vi "Prompt for App Instance.vi"(8 "error in (no error)":errorcluster, 10 "Calling VI in":refnum<vi>, 11 "App Instances":T1[](array[typedef])) -> (0 "error out":errorcluster, 2 "OK?":bool, 3 "App Ref":refnum<vi>)   [LabVIEW 2020, in "MacroAssert.lvlib"]
doc: "Displays a window to select the application instance to connect to."
uses:
  MacroAssert.lvlib
  FaKI State Machine/FaKI State Machine.lvlib
  CTLs/FGV Actions.ctl
  Custom Errors/Custom Errors.lvlib
  <vilib>/Utility/miscctls.llb/LVComboBoxStrsAndValuesArrayTypeDef.ctl
  CTLs/App Instance.ctl
  <userlib>/_MGI/Application Control/MGI Gray if/MGI Gray if False.vi
panel:
  in  "Project":string(combo)
  in  "App Instance":string(combo)
  in  "OK":bool
  in  "Exit":bool
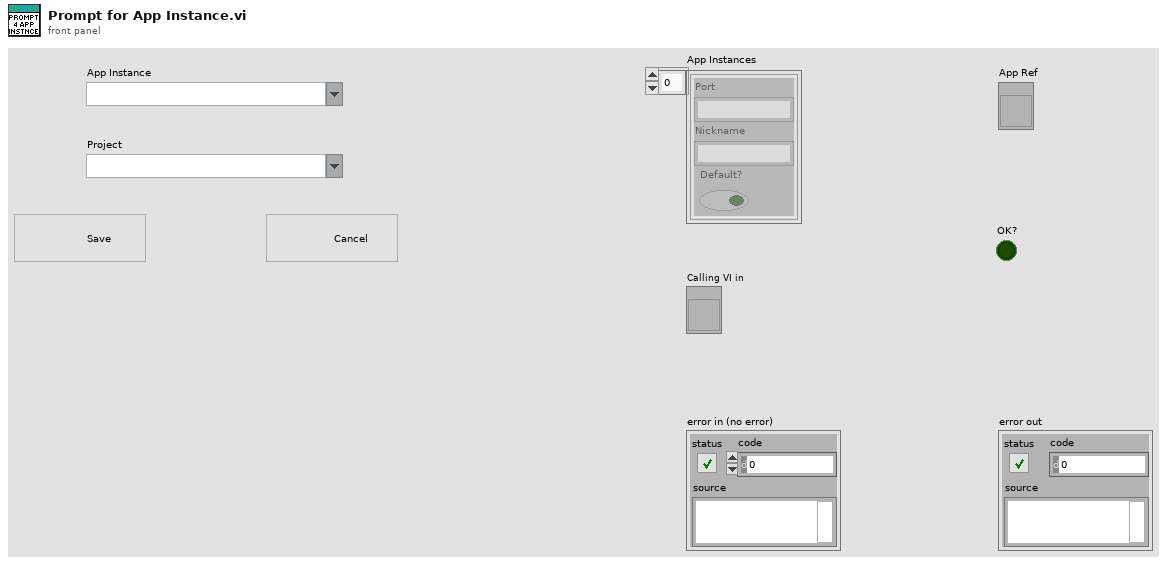
[diagram p1: front panel]
types:
  T1 = typedef "MacroAssert.lvlib/App Instance.ctl" = cluster{"Port":string, "Nickname":string, "Default?":bool}
  T2 = enum32{"Invalid", "Standard", "Closed", "Hidden", "Minimized", "Maximized"}
  T3 = enum32{"invalid app kind", "Development System", "Run Time System", "Student Edition", "Embedded LabVIEW", "Evaluation", "Custom"}
  T4 = typedef "LVComboBoxStrsAndValuesArrayTypeDef.ctl" = cluster{"String":string, "Value":string}[]
  T5 = typedef "MacroAssert.lvlib/FGV Actions.ctl" = enum16{"Read", "Write"}
  T6 = cluster{"Core":cluster{"Current VI Reference":refnum<vi>, "Close Panel on Exit?":bool}, "App Instances":T1[], "Current App":T1, "Current Proj":path, "App Ref":refnum<vi>, "Projects":cluster{"Name":string, "Path":path}[], "OK?":bool}
  T7 = cluster{"Current VI Reference":refnum<vi>, "Close Panel on Exit?":bool}
  T8 = enum8{"Enabled", "Disabled", "Disabled and Grayed Out"}
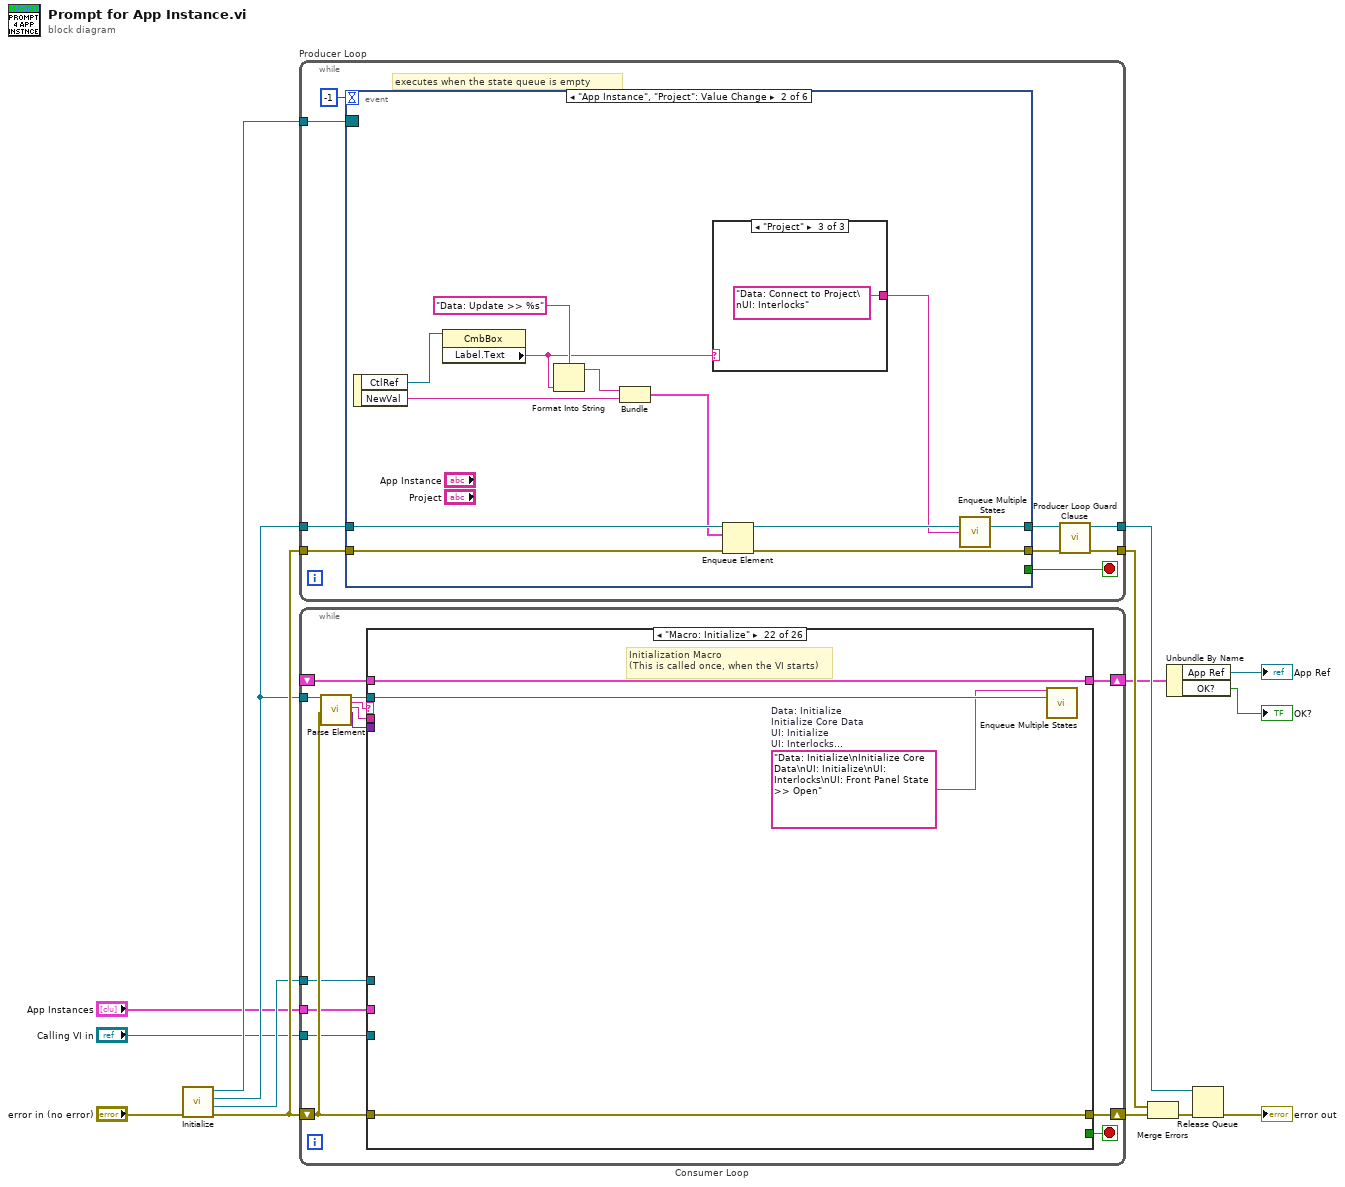
[diagram p0: block diagram]
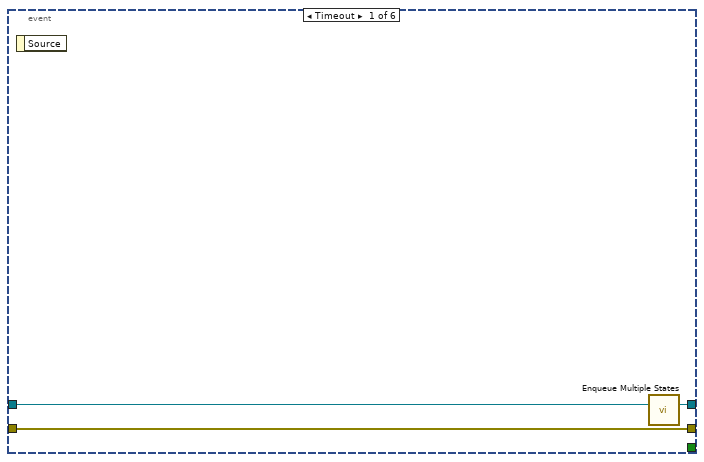
[diagram p2: hidden frame]
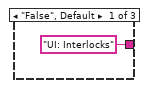
[diagram p3: hidden frame]
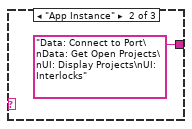
[diagram p4: hidden frame]
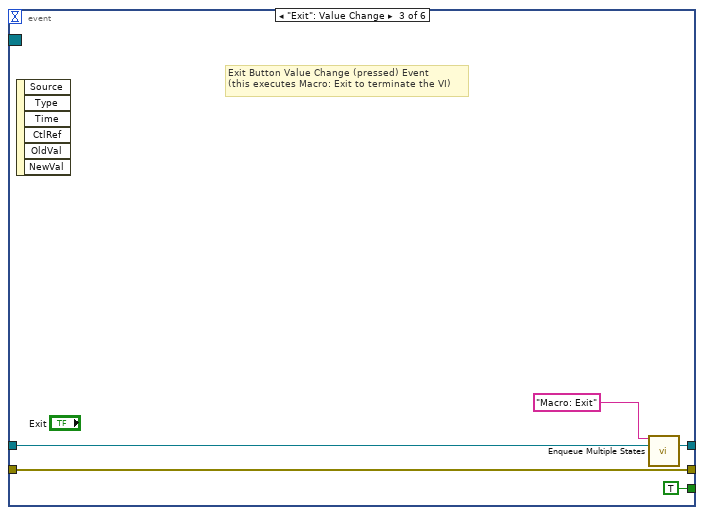
[diagram p5: hidden frame]
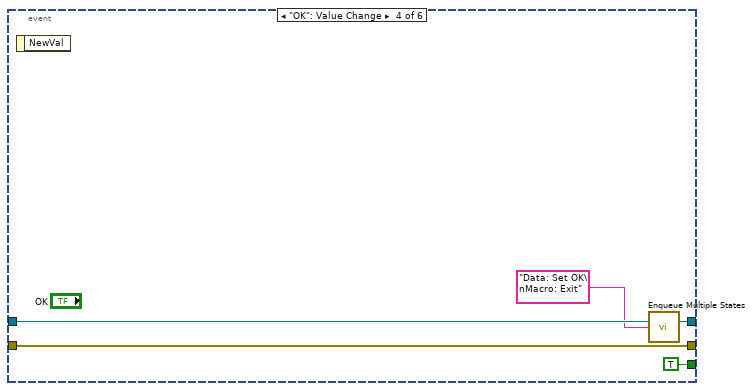
[diagram p6: hidden frame]
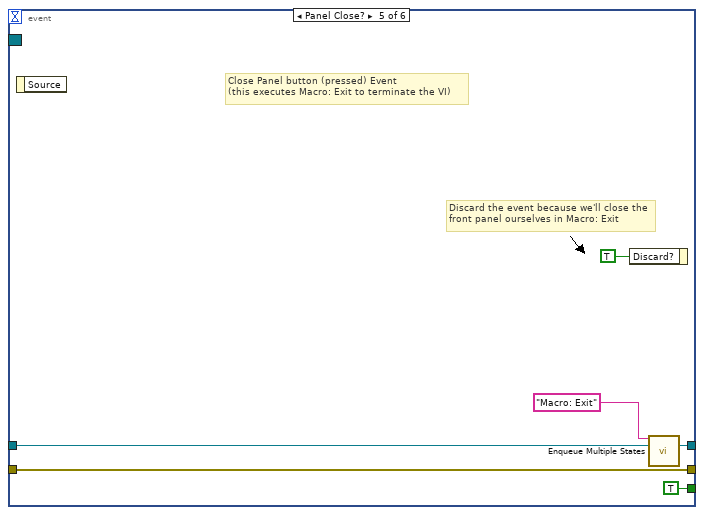
[diagram p7: hidden frame]
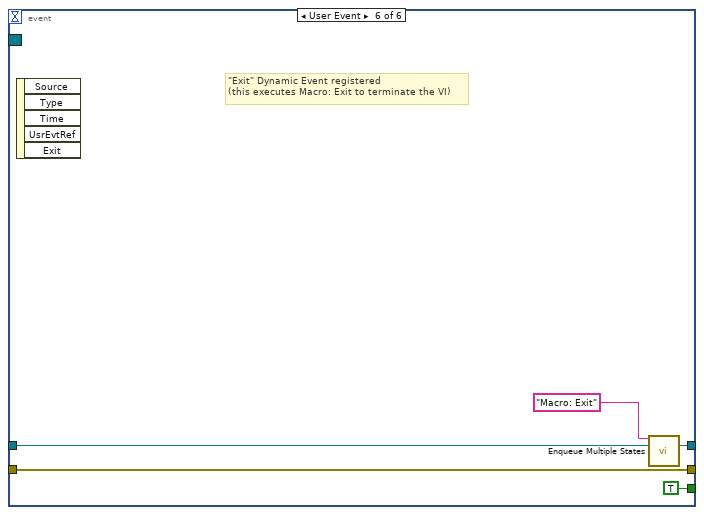
[diagram p8: hidden frame]
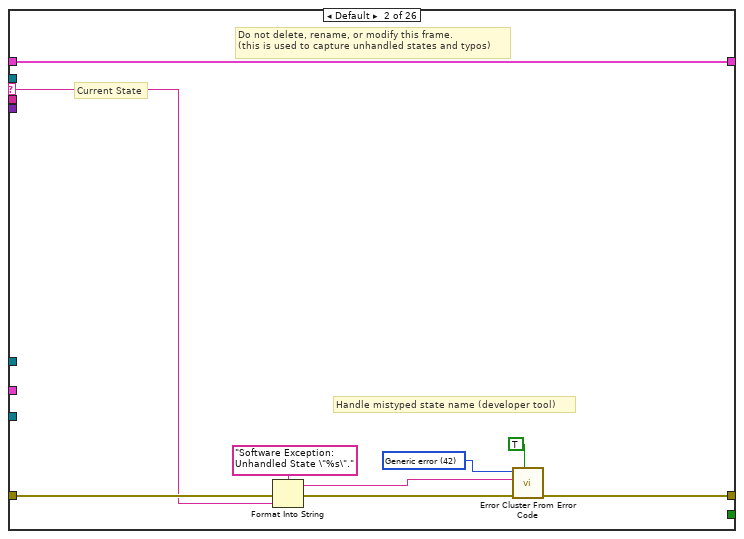
[diagram p10: hidden frame]
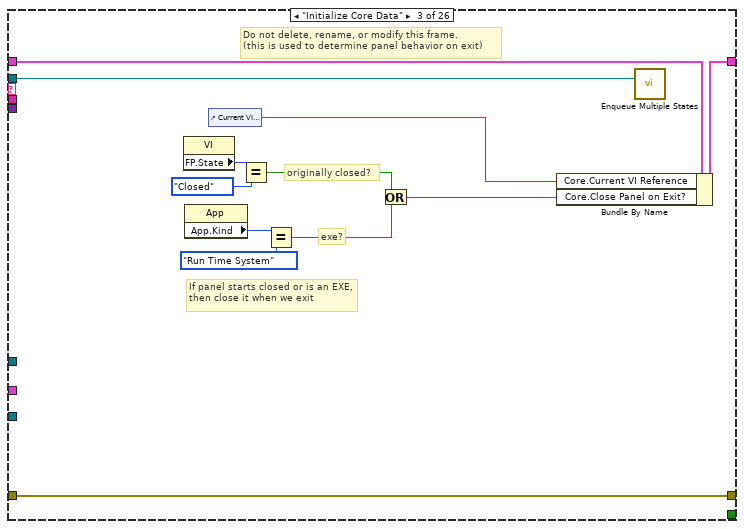
[diagram p11: hidden frame]
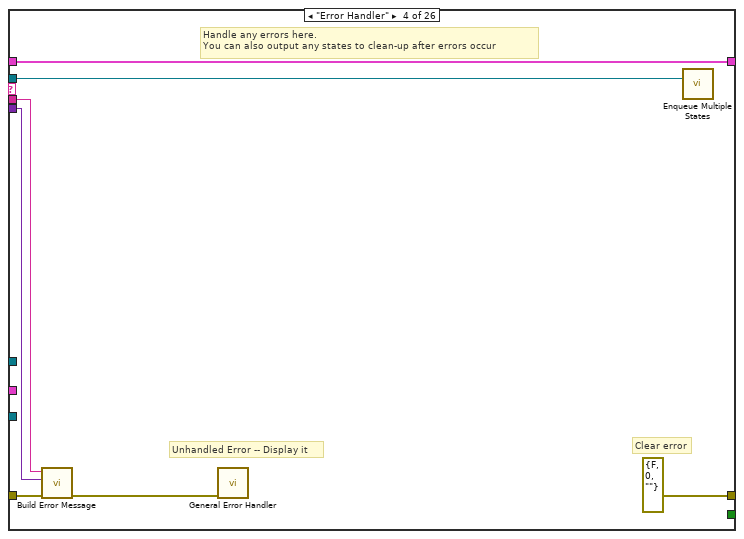
[diagram p12: hidden frame]
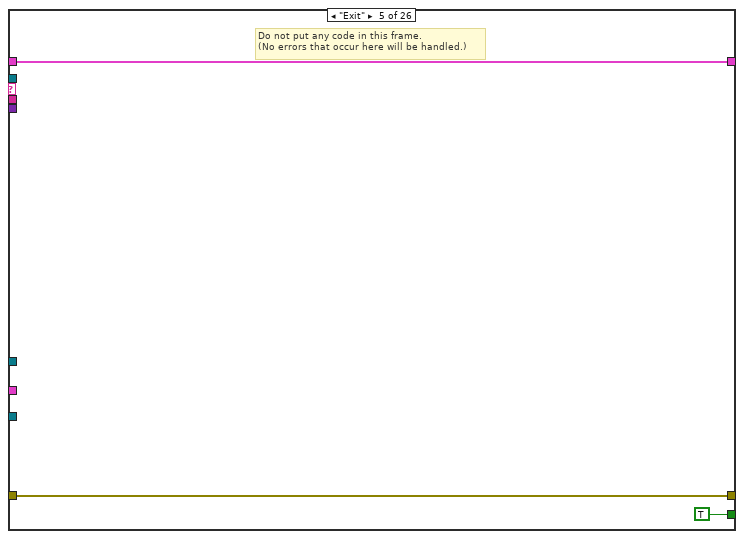
[diagram p13: hidden frame]
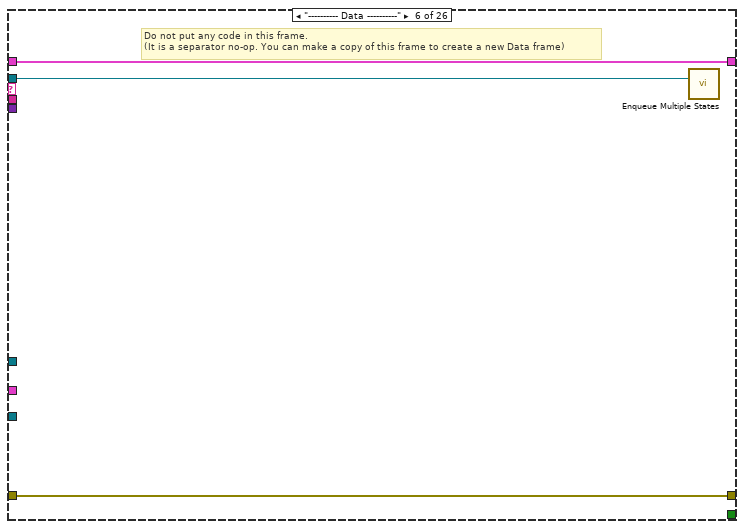
[diagram p14: hidden frame]
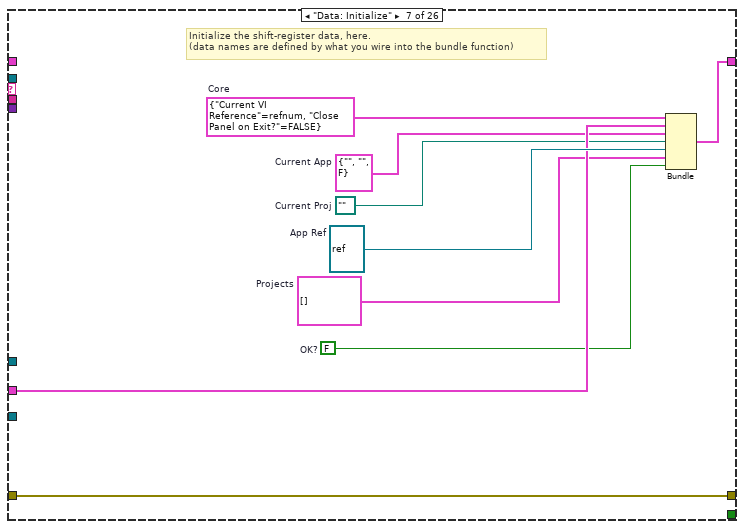
[diagram p15: hidden frame]
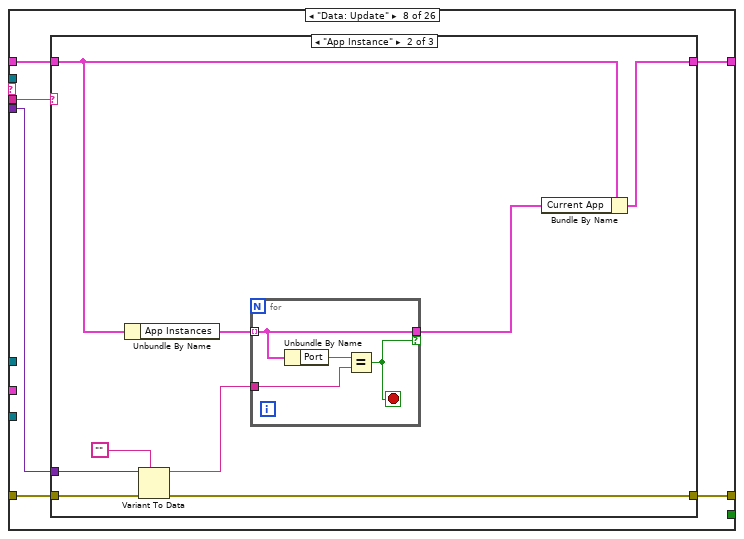
[diagram p16: hidden frame]
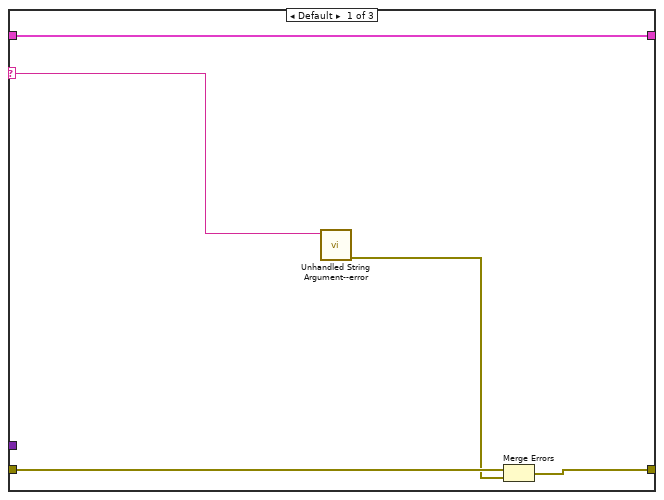
[diagram p17: hidden frame]
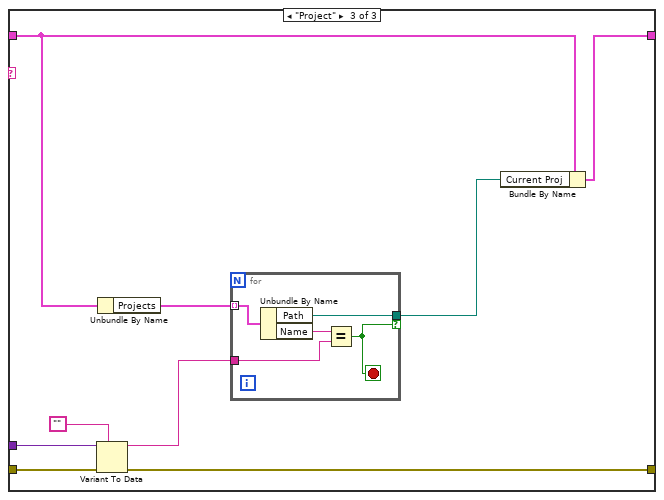
[diagram p18: hidden frame]
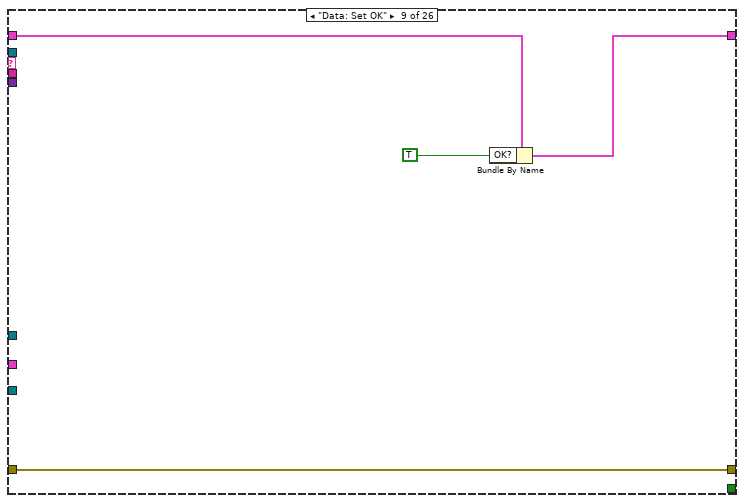
[diagram p19: hidden frame]
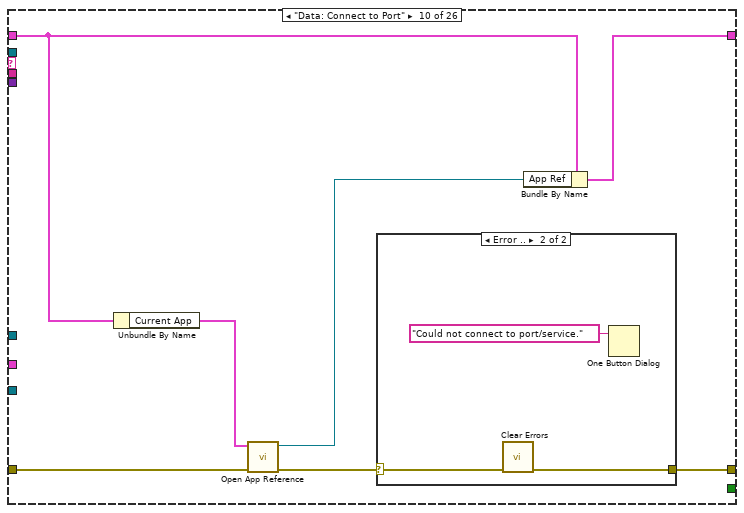
[diagram p20: hidden frame]
diagram:
  n1 = call "Initialize.vi"("error in (no error)"="error in (no error)") -> ("error out"=w11:errorcluster, "Exit Event"=w8:refnum<user-event>, "Queue"=w7:refnum<queue>, "Event Registration Refnum"=w6:refnum<event-registration>)  [unwired: 7 in]
  n2 = while "Producer Loop" {
    tunnel: w6 -> [w18]
    tunnel: w7 -> [w21]
    tunnel: [w19] -> w9
    tunnel: w11 -> [w24]
    tunnel: [w22] -> w14
    stop <- w16 stop-if-true
    # "executes when the state queue is empty"
    n3 = event shown="[1] \"App Instance\", \"Project\": Value Change" {
      selector: w18 -> [_ _ _ _ _ _]
      dyn-events: _ -> [_ _ _ _ _ _]
      timeout: -1 ("Timeout") -> [_ _ _ _ _ _]
      tunnel: [w27 w38 w47 w52 w58 w63] -> w23
      tunnel: w24 -> [w27 w39 w47 w52 w58 w63]
      tunnel: w21 -> [w25 w37 w46 w51 w57 w62]
      tunnel: [w26 w34 w45 w50 w56 w61] -> w20
      tunnel: [_ _ TRUE TRUE TRUE TRUE] -> w16
      event Timeout {
        n4 = event-data() -> ()  [unwired: 1 in, 1 out]
        n5 = call "Enqueue Multiple States.vi"("queue in"=w25) -> ("queue out"=w26:refnum<queue>)  [unwired: 14 in]
      }
      event "App Instance", "Project": Value Change {
        n6 = event-data() -> ("CtlRef"=w35:refnum<vi>, "NewVal"=w28:string)  [unwired: 1 in]
        n7 = property class="CmbBox"(reference=w35) -> ("Label.Text"=w30:string)  [unwired: 1 in, 2 out]
        n8 = Format Into String(format string="Data: Update >> %s", w30) -> (resulting string=w31:string)  [unwired: 2 in, 1 out]
        n9 = Bundle(w31, "NewVal"=w28) -> (w29:cluster{string, "NewVal":string})  [unwired: 1 in]
        n10 = case shown="\"Project\"" w30 {
          tunnel: ["UI: Interlocks" ("string") "Data: Connect to Port\nData: Get Open Projects\nUI: Display Projects\nUI: Interlocks" ("string") "Data: Connect to Project\nUI: Interlocks" ("string")] -> w33
          frame "False", Default {
          }
          frame "App Instance" {
          }
          frame "Project" {
          }
        }
        n11 = Enqueue Element(queue=w37, element=w29, error in (no error)=w39) -> (queue out=w36:refnum<queue>, error out=w38:errorcluster)  [unwired: 1 in, 1 out]
        n12 = call "Enqueue Multiple States.vi"("queue in"=w36, "State(s) at Back"=w33) -> ("queue out"=w34:refnum<queue>)  [unwired: 13 in]
      }
      event "Exit": Value Change {
        # "Exit Button Value Change (pressed) Event\n(this executes Macro: Exit to terminate the VI)"
        n13 = event-data() -> ()  [unwired: 1 in, 6 out]
        n14 = call "Enqueue Multiple States.vi"("State(s) at Front"="Macro: Exit", "queue in"=w46) -> ("queue out"=w45:refnum<queue>)  [unwired: 13 in]
      }
      event "OK": Value Change {
        n15 = event-data() -> ()  [unwired: 1 in, 1 out]
        n16 = call "Enqueue Multiple States.vi"("queue in"=w51, "State(s) at Back"="Data: Set OK\nMacro: Exit") -> ("queue out"=w50:refnum<queue>)  [unwired: 13 in]
      }
      event Panel Close? {
        # "Discard the event because we'll close the front panel ourselves in Macro: Exit"
        # "Close Panel button (pressed) Event\n(this executes Macro: Exit to terminate the VI)"
        n17 = event-data() -> ()  [unwired: 1 in, 1 out]
        n18 = event-data("Discard?"=TRUE) -> ()  [unwired: 1 in, 1 out]
        n19 = call "Enqueue Multiple States.vi"("State(s) at Front"="Macro: Exit", "queue in"=w57) -> ("queue out"=w56:refnum<queue>)  [unwired: 13 in]
      }
      event User Event {
        # "\"Exit\" Dynamic Event registered\n(this executes Macro: Exit to terminate the VI)"
        n20 = event-data() -> ()  [unwired: 1 in, 5 out]
        n21 = call "Enqueue Multiple States.vi"("State(s) at Front"="Macro: Exit", "queue in"=w62) -> ("queue out"=w61:refnum<queue>)  [unwired: 13 in]
      }
    }
    n22 = call "Producer Loop Guard Clause.vi"("error in (no error)"=w23, "queue in"=w20) -> ("error out"=w22:errorcluster, "queue out"=w19:refnum<queue>)  [unwired: 8 in]
  }
  n23 = while "Consumer Loop" {
    shift-right: [w69] -> w3
    shift-left: _ -> [w68]
    shift-right: [w76] -> w13
    shift-left: w11 -> [w75]
    tunnel: w7 -> [w74]
    tunnel: w8 -> [w72]
    tunnel: "App Instances" -> [w64]
    tunnel: "Calling VI in" -> [w71]
    stop <- w70 stop-if-true
    n24 = call "Parse Element.vi"("queue in"=w74, "error in (no error)"=w75) -> ("queue out"=w73:refnum<queue>, "State"=w67:string, "Arg"=w66:string, "Data"=w65:variant)  [unwired: 14 in]
    n25 = case shown="\"Macro: Initialize\"" w67 {
      selector: w67 -> [_ w79 _ _ _ _ _ _ _ _ _ _ _ _ _ _ _ _ _ _ _ _ _ _ _ _]
      tunnel: w73 -> [_ _ w97 w103 _ w111 _ _ _ _ _ _ _ _ _ _ _ _ _ _ _ w348 w358 _ _ w373]
      tunnel: w66 -> [_ _ _ w100 _ _ _ w125 _ _ _ _ _ _ _ _ w227 w235 _ _ _ _ _ _ _ _]
      tunnel: w68 -> [w77 w81 w92 w102 w108 w110 _ w124 w162 w165 w176 w188 w208 w212 w216 w225 w228 w236 w314 w340 w344 w347 w357 w360 w364 w372]
      tunnel: [w78 w86 w99 errorcluster {"status"=FALSE, "code"=0, "source"=""} ("error out") w109 w112 w121 w126 w163 w168 w180 w189 w210 w213 w217 w226 w229 w239 w318 w341 w345 w349 w359 w361 w365 w374] -> w76
      tunnel: w75 -> [w78 w85 w99 w105 w109 w112 w121 w127 w163 w170 w182 w190 w211 w213 w217 w226 w230 w240 w317 w341 w345 w349 w359 w361 w366 w375]
      tunnel: [_ _ _ _ TRUE _ _ _ _ _ _ _ _ _ _ _ _ _ _ _ _ _ _ _ _ _] -> w70
      tunnel: [w77 w81 w96 w102 w108 w110 w119 w122 w161 w166 w177 w187 w208 w212 w216 w225 w228 w236 w314 w340 w344 w347 w357 w360 w364 w372] -> w69
      tunnel: w65 -> [_ _ _ w101 _ _ _ w123 _ _ _ _ _ _ _ _ _ _ _ _ _ _ _ _ _ _]
      tunnel: w72 -> [_ _ _ _ _ _ _ _ _ _ _ _ _ _ _ _ _ _ _ _ _ _ _ _ _ _]
      tunnel: w64 -> [_ _ _ _ _ _ w117 _ _ _ _ _ _ _ _ _ _ _ _ _ _ _ _ _ _ _]
      tunnel: w71 -> [_ _ _ _ _ _ _ _ _ _ _ _ _ _ _ _ _ w237 _ _ _ _ _ _ _ _]
      frame "---------- Core ----------" {
        # "Do not put any code in this frame.\n(it is a separator no-op)"
      }
      frame Default {
        w83 = 42 items=["No error", "Argument error", "Memory is full", "Out of zone", "End of file", "File already open", "Generic file I/O error", "File not found", "File permission error", "Disk is full", "Duplicate path", "Too many files open", "System feature not enabled", "Resource file not found", "Cannot add resource", "Resource not found", "Image not found", "Image memory error", "Pen does not exist", "Config type invalid", "Config token not found", "Config parse error", "Config memory error", "Bad external code format", "Bad external code offset", "External code not present", "Null window", "Destroy window error", "Null menu", "Print aborted", "Bad print record", "Print driver error", "Windows error during printing", "Memory error during printing", "Print dialog error", "Generic print error", "Invalid device refnum", "Device not found", "Device parameter error", "Device unit error", "Cannot open device", "Device call aborted", "Generic error", "Cancelled by user", "Object ID too low", "Object ID too high", "Object not in heap", "Unknown heap", "Unknown object (invalid DefProc)", "Unknown object (DefProc not in table)", "Message out of range", "Invalid (null) method", "Unknown message", "Manager call not supported", "Bad address", "Network operation in progress", "Network operation timed out", "Connection is busy", "Network attribute not supported", "Network error", "Address in use", "System out of memory", "Connection aborted", "Connection refused", "Not connected", "Already connected", "Connection closed", "Initialization error (interapplication manager)", "Bad occurrence", "Wait on unbound occurrence handler", "Occurrence queue overflow", "Datalog type conflict", "Unused", "Unrecognized type (interapplication manager)", "Memory corrupt", "Failed to make temporary DLL", "Old CIN version", "Drag socket not found", "Failed to load drop-object", "Failed to register OLE object", "Failed to release OLE object", "Format specifier type mismatch", "Unknown format specifier", "Too few format specifiers", "Too many format specifiers", "Scan failed", "Newer CIN version", "Error converting to variant", "Runtime menu error", "Password tampered", "Variant attribute not found", "Incompatible variant data type", "Event data is not available", "Event Store is not present", "Occurrence is not found", "Event Queue is not created", "Event info is not available", "Refnum passed is NULL", "Error retrieving Class GUID", "Error retrieving CoClass GUID", "Error retrieving TypeLib GUID.", "Bad built application magic bytes.", "Specific driver is different from the specific driver associated with the Logical Name.", "There is no session opened to the class driver.", "Max Error", "MAX - Error with config objects", "MAX - Error loading configuration", "MAX - Group not supported"]
        # "Current State"
        # "Do not delete, rename, or modify this frame.\n(this is used to capture unhandled states and typos)"
        # "Handle mistyped state name (developer tool)"
        n26 = Format Into String(format string="Software Exception: Unhandled State \"%s\"." ("message"), error in=w85, w79) -> (resulting string=w82:string, error out=w87:errorcluster)  [unwired: 1 in]
        n27 = call <vilib>:"Error Cluster From Error Code.vi"("show call chain? (False)"=TRUE, "error in (no error)"=w87, "error message (\"\")"=w82, "error code (0)"=w83) -> ("error out"=w86:errorcluster)  [unwired: 5 in]
      }
      frame "Initialize Core Data" {
        # "Do not delete, rename, or modify this frame.\n(this is used to determine panel behavior on exit)"
        # "originally closed?"
        # "exe?"
        # "If panel starts closed or is an EXE, then close it when we exit"
        n28 = property class="VI"() -> ("FP.State"=w90:T2)  [unwired: 2 in, 2 out]
        n29 = property class="App"() -> ("App.Kind"=w95:T3)  [unwired: 2 in, 2 out]
        n30 = control-ref of="Current VI Reference"() -> (w98:refnum<vi>)
        n31 = Equal?(x=w90, y=T2."Closed" ("Front Panel Window:State")) -> (x = y?=w88:bool)
        n32 = Equal?(x=w95, y=T3."Run Time System" ("Application:Kind")) -> (x = y?=w93:bool)
        n33 = Or(x=w88, y=w93) -> (x .or. y?=w91:bool)
        n34 = Bundle By Name(cluster=w92, "Core.Current VI Reference"=w98, "Core.Close Panel on Exit?"=w91) -> (w96:T6)
        n35 = call "Enqueue Multiple States.vi"("queue in"=w97) -> ()  [unwired: 14 in, 1 out]
      }
      frame "Error Handler" {
        # "Unhandled Error -- Display it"
        # "Handle any errors here.\nYou can also output any states to clean-up after errors occur"
        # "Clear error"
        n36 = call "Build Error Message.vi"("error in (no error)"=w105, "Data"=w101, "Arg"=w100) -> ("error out"=w104:errorcluster)  [unwired: 8 in]
        n37 = call <vilib>:"General Error Handler.vi"("error in (no error)"=w104) -> ()  [unwired: 10 in, 5 out]
        n38 = call "Enqueue Multiple States.vi"("queue in"=w103) -> ()  [unwired: 14 in, 1 out]
      }
      frame "Exit" {
        # "Do not put any code in this frame.\n(No errors that occur here will be handled.)"
      }
      frame "---------- Data ----------" {
        # "Do not put any code in this frame.\n(It is a separator no-op. You can make a copy of this frame to create a new Data frame)"
        n39 = call "Enqueue Multiple States.vi"("queue in"=w111) -> ()  [unwired: 14 in, 1 out]
      }
      frame "Data: Initialize" {
        w113 = path ""  # Current Proj
        w114 = T1 {"Port"="", "Nickname"="", "Default?"=FALSE}  # Current App
        w115 = cluster{"Name":string, "Path":path}[] []  # Projects
        w120 = refnum<vi> refnum  # App Ref
        w116 = FALSE  # OK?
        w118 = T7 {"Current VI Reference"=refnum, "Close Panel on Exit?"=FALSE}  # Core
        # "Initialize the shift-register data, here.\n(data names are defined by what you wire into the bundle function)"
        n40 = Bundle("Core"=w118, "App Instances"=w117, "Current App"=w114, "Current Proj"=w113, "App Ref"=w120, "Projects"=w115, "OK?"=w116) -> (w119:T6)  [unwired: 1 in]
      }
      frame "Data: Update" {
        n41 = case shown="\"App Instance\"" w125 {
          selector: w125 -> [w129 _ _]
          tunnel: w124 -> [w128 w136 w149]
          tunnel: w127 -> [w132 w141 w154]
          tunnel: w123 -> [_ w139 w152]
          tunnel: [w130 w140 w153] -> w126
          tunnel: [w128 w137 w150] -> w122
          frame Default {
            n42 = call "Unhandled String Argument--error.vi"("Argument"=w129) -> ("error out"=w131:errorcluster)  [unwired: 10 in]
            n43 = Merge Errors(w132, w131) -> (w130:errorcluster)
          }
          frame "App Instance" {
            n44 = Unbundle By Name(w136) -> ("App Instances"=w135:T1[])
            n45 = Variant To Data(error in=w141, type="", Variant=w139) -> (data=w134:string, error out=w140:errorcluster)
            n46 = for {
              tunnel: w135 -> [w143] mode=indexing
              tunnel: w134 -> [w144]
              tunnel: [w143] -> w133 if=w142
              stop <- w142 stop-if-true
              n47 = Unbundle By Name(w143) -> ("Port"=w145:string)
              n48 = Equal?(x=w145, y=w144) -> (x = y?=w142:bool)
            }
            n49 = Bundle By Name(cluster=w136, "Current App"=w133) -> (w137:T6)
          }
          frame "Project" {
            n50 = Variant To Data(error in=w154, type="", Variant=w152) -> (data=w147:string, error out=w153:errorcluster)
            n51 = Unbundle By Name(w149) -> ("Projects"=w148:cluster{"Name":string, "Path":path}[])
            n52 = for {
              tunnel: w148 -> [w157] mode=indexing
              tunnel: w147 -> [w158]
              tunnel: [w155] -> w146 if=w156
              stop <- w156 stop-if-true
              n53 = Unbundle By Name(w157) -> ("Path"=w155:path, "Name"=w159:string)
              n54 = Equal?(x=w159, y=w158) -> (x = y?=w156:bool)
            }
            n55 = Bundle By Name(cluster=w149, "Current Proj"=w146) -> (w150:T6)
          }
        }
      }
      frame "Data: Set OK" {
        n56 = Bundle By Name(cluster=w162, "OK?"=TRUE) -> (w161:T6)
      }
      frame "Data: Connect to Port" {
        n57 = Unbundle By Name(w165) -> ("Current App"=w164:T1)
        n58 = call "Open App Reference.vi"("error in (no error)"=w170, "App Instance"=w164) -> ("error out"=w169:errorcluster, "App Ref"=w167:refnum<vi>)  [unwired: 8 in]
        n59 = case shown="Error .." w169 {
          selector: w169 -> [w171 w174]
          tunnel: [w171 w173] -> w168
          frame No Error {
          }
          frame Error {
            n60 = call <vilib>:"Clear Errors.vi"("error in (no error)"=w174) -> ("error out"=w173:errorcluster)  [unwired: 5 in, 1 out]
            n61 = One Button Dialog(message="Could not connect to port/service.") -> ()  [unwired: 1 in, 1 out]
          }
        }
        n62 = Bundle By Name(cluster=w165, "App Ref"=w167) -> (w166:T6)
      }
      frame "Data: Connect to Project" {
        n63 = Unbundle By Name(w176) -> ("App Ref"=w178:refnum<vi>, "Current Proj"=w175:path)
        n64 = call "Open Project Reference.vi"("error in (no error)"=w182, "Path"=w175, "App Ref"=w178) -> ("error out"=w181:errorcluster, "App Ref out"=w179:refnum<vi>)  [unwired: 7 in]
        n65 = case shown="Error .." w181 {
          selector: w181 -> [w183 w186]
          tunnel: [w183 w185] -> w180
          frame No Error {
          }
          frame Error {
            n66 = call <vilib>:"Clear Errors.vi"("error in (no error)"=w186) -> ("error out"=w185:errorcluster)  [unwired: 5 in, 1 out]
            n67 = One Button Dialog(message="Could not connect to port/service.") -> ()  [unwired: 1 in, 1 out]
          }
        }
        n68 = Bundle By Name(cluster=w176, "App Ref"=w179) -> (w177:T6)
      }
      frame "Data: Get Open Projects" {
        n69 = in-place {
          in-place-border: w190 -> [w198]
          in-place-border: [w199] -> w189
          n70 = in-place-cluster #1(w188) -> ("App Ref"=w196:refnum<vi>)  [unwired: 1 out]
          n71 = property class="App"(reference=w196) -> (reference out=w195:refnum<vi>, error out=w200:errorcluster, "Project"=w194:refnum<vi>[])  [unwired: 1 in]
          n72 = for {
            tunnel: w200 -> [w207]
            tunnel: w194 -> [w205] mode=indexing
            tunnel: [w206] -> w192 mode=indexing
            tunnel: [w204] -> w193 mode=indexing
            tunnel: [w201] -> w191 mode=indexing
            n73 = property class="Project"(reference=w205, error in=w207) -> (reference out=w204:refnum<vi>, error out=w206:errorcluster, "Name"=w202:string, "Path"=w203:path)
            n74 = Bundle("Name"=w202, "Path"=w203) -> (w201:cluster{"Name":string, "Path":path})  [unwired: 1 in]
          }
          n75 = Close Reference(reference=w193) -> (error out=w197:errorcluster)  [unwired: 1 in]
          n76 = Merge Errors(w198, w197, w192) -> (w199:errorcluster)
          n77 = in-place-cluster #1("App Ref"=w195, "Projects"=w191) -> (w187:T6)
        }
      }
      frame "Data: Cleanup" {
        # "Cleanup any data and references, here.\n(this is called automatically, by the Macro: Exit)"
        n78 = Unbundle By Name(w208) -> ("Core.Current VI Reference"=w209:refnum<vi>)
        n79 = Close Reference(reference=w209, error in (no error)=w211) -> (error out=w210:errorcluster)
      }
      frame "---------- UI ----------" {
        # "Do not put any code in this frame.\n(It is a separator no-op. You can make a copy of this frame to create a new UI frame)"
      }
      frame "UI: Initialize" {
        # "Initialize the User Interface, here.\n(this is called automatically, by the Macro: Init)"
        n80 = Unbundle By Name(w216) -> ("App Instances"=w215:T1[])
        n81 = for {
          tunnel: w215 -> [w221] mode=indexing
          tunnel: [w218] -> w214 mode=indexing
          n82 = Unbundle By Name(w221) -> ("Nickname"=w220:string, "Port"=w219:string)
          n83 = Bundle("Nickname"=w220, "Port"=w219) -> (w218:cluster{"Nickname":string, "Port":string})  [unwired: 1 in]
        }
        n84 = property on="App Instance" class="CmbBox"("Strings And Values[]"=w214) -> ()  [unwired: 2 in, 2 out]
      }
      frame "UI: Uninitialize" {
        w222 = ""
        # "Uninitialize the User Interface, here.\n(this is called automatically, by the Macro: Exit)"
        n85 = property on="App Instance" class="CmbBox"("Strings And Values[]"=T4 [] ("Strings And Values []"), "Value"=w222) -> ()  [unwired: 2 in, 2 out]
        n86 = property on="Project" class="CmbBox"("Strings And Values[]"=T4 [] ("Strings And Values []"), "Value"=w222) -> ()  [unwired: 2 in, 2 out]
      }
      frame "UI: Cursor Set" {
        # "Argument"
        # "Set and Unset Cursor Busy.\n(Usage: \"UI: Cursor Set >> Busy|Idle\")"
        n87 = case shown="\"Idle\", Default" w227 {
          tunnel: w230 -> [w232 w234]
          tunnel: [w231 w233] -> w229
          frame "Idle", Default {
            n88 = call <vilib>:"Unset Busy.vi"("error in (no error)"=w232) -> ("error out"=w231:errorcluster)  [unwired: 10 in]
          }
          frame "Busy" {
            n89 = call <vilib>:"Set Busy.vi"("error in (no error)"=w234) -> ("error out"=w233:errorcluster)  [unwired: 9 in, 1 out]
          }
        }
      }
      frame "UI: Front Panel State" {
        # "Argument"
        # "Set Front Panel Open or Closed\n(Usage: \"UI: Front Panel State >> Open|Close\")"
        n90 = Unbundle By Name(w236) -> ("Core.Current VI Reference"=w238:refnum<vi>)
        n91 = case shown="\"Open\", \"Standard\", Default" w235 {
          tunnel: w240 -> [w248 w265 w277 w290 w303]
          tunnel: [w249 w266 w278 w291 w304] -> w239
          tunnel: w238 -> [w246 w263 w275 w288 w301]
          tunnel: w237 -> [w244 _ _ _ _]
          frame "Open", "Standard", Default {
            w241 = T2."Standard" ("State")
            n92 = property class="VI"(reference=w246, error in=w248) -> (reference out=w245:refnum<vi>, error out=w247:errorcluster, "FP.State"=w243:T2)
            n93 = Not Equal?(x=w243, y=w241) -> (x != y?=w242:bool)
            n94 = case shown="True" w242 {
              tunnel: [w257 w258] -> w249
              tunnel: w247 -> [w256 w258]
              tunnel: w245 -> [w254 _]
              tunnel: w241 -> [w250 _]
              tunnel: w244 -> [w252 _]
              frame True {
                n95 = call "Center Dialog on Caller.vi"("error in (no error)"=w256, "Dialog VI"=w254, "Calling VI in"=w252) -> ("error out"=w255:errorcluster, "Dialog VI out"=w253:refnum<vi>)  [unwired: 7 in]
                n96 = invoke class="VI" method="FP.Open"(reference=w253, error in=w255, "Activate"=TRUE, "State"=w250) -> (error out=w257:errorcluster)  [unwired: 1 in, 4 out]
              }
              frame False {
              }
            }
          }
          frame "Close", "Closed" {
            n97 = property class="VI"(reference=w263, error in=w265) -> (reference out=w262:refnum<vi>, error out=w264:errorcluster, "FP.State"=w260:T2)
            n98 = Not Equal?(x=w260, y=T2."Closed" ("Front Panel Window:State")) -> (x != y?=w259:bool)
            n99 = case shown="True" w259 {
              tunnel: [w267 w270] -> w266
              tunnel: w264 -> [w267 w269]
              tunnel: w262 -> [_ w268]
              frame False {
              }
              frame True {
                n100 = invoke class="VI" method="FP.Close"(reference=w268, error in=w269) -> (error out=w270:errorcluster)  [unwired: 1 in, 2 out]
              }
            }
          }
          frame "Hidden", "Hide" {
            w271 = T2."Hidden" ("State")
            n101 = property class="VI"(reference=w275, error in=w277) -> (reference out=w274:refnum<vi>, error out=w276:errorcluster, "FP.State"=w273:T2)
            n102 = Not Equal?(x=w273, y=w271) -> (x != y?=w272:bool)
            n103 = case shown="True" w272 {
              tunnel: [w282 w283] -> w278
              tunnel: w276 -> [w281 w283]
              tunnel: w274 -> [w280 _]
              tunnel: w271 -> [w279 _]
              frame True {
                n104 = invoke class="VI" method="FP.Open"(reference=w280, error in=w281, "State"=w279) -> (error out=w282:errorcluster)  [unwired: 2 in, 4 out]
              }
              frame False {
              }
            }
          }
          frame "Minimize", "Minimized" {
            w284 = T2."Minimized" ("State")
            n105 = property class="VI"(reference=w288, error in=w290) -> (reference out=w287:refnum<vi>, error out=w289:errorcluster, "FP.State"=w286:T2)
            n106 = Not Equal?(x=w286, y=w284) -> (x != y?=w285:bool)
            n107 = case shown="True" w285 {
              tunnel: [w295 w296] -> w291
              tunnel: w289 -> [w294 w296]
              tunnel: w287 -> [w293 _]
              tunnel: w284 -> [w292 _]
              frame True {
                n108 = invoke class="VI" method="FP.Open"(reference=w293, error in=w294, "State"=w292) -> (error out=w295:errorcluster)  [unwired: 2 in, 4 out]
              }
              frame False {
              }
            }
          }
          frame "Maximize", "Maximized" {
            w297 = T2."Maximized" ("State")
            n109 = property class="VI"(reference=w301, error in=w303) -> (reference out=w300:refnum<vi>, error out=w302:errorcluster, "FP.State"=w299:T2)
            n110 = Not Equal?(x=w299, y=w297) -> (x != y?=w298:bool)
            n111 = case shown="True" w298 {
              tunnel: [w308 w309] -> w304
              tunnel: w302 -> [w307 w309]
              tunnel: w300 -> [w306 _]
              tunnel: w297 -> [w305 _]
              frame True {
                n112 = invoke class="VI" method="FP.Open"(reference=w306, error in=w307, "State"=w305) -> (error out=w308:errorcluster)  [unwired: 2 in, 4 out]
              }
              frame False {
              }
            }
          }
        }
      }
      frame "UI: Interlocks" {
        n113 = Unbundle By Name(w314) -> ("App Ref"=w316:refnum<vi>)
        n114 = property class="App"(reference=w316, error in=w317) -> (reference out=w315:refnum<vi>, error out=w319:errorcluster, "App.Kind"=w313:T3)
        n115 = case shown="\"Development System\"" w313 {
          tunnel: w315 -> [_ w329 _]
          tunnel: w319 -> [w323 w333 w336]
          tunnel: [w322 w330 w336] -> w318
          tunnel: [FALSE w326 TRUE] -> w312
          tunnel: [FALSE TRUE FALSE] -> w310
          frame "invalid app kind", Default {
            n116 = call <vilib>:"Clear Errors.vi"("error in (no error)"=w323) -> ("error out"=w322:errorcluster)  [unwired: 5 in, 1 out]
          }
          frame "Development System" {
            n117 = property class="App"(reference=w329, error in=w333) -> (error out=w332:errorcluster, "Project.OwningProject"=w328:refnum<vi>)  [unwired: 1 out]
            n118 = property class="Project" props=["Name"](reference=w328, error in=w332) -> (error out=w331:errorcluster)  [unwired: 2 out]
            n119 = call <vilib>:"Clear Errors.vi"("error in (no error)"=w331, "specific error code to clear (0: all)"=56004) -> ("error out"=w330:errorcluster, "specific error cleared?"=w324:bool)  [unwired: 4 in]
            n120 = Not(x=w324) -> (.not. x?=w326:bool)
          }
          frame "Run Time System" {
          }
        }
        n121 = call-poly <userlib>:"MGI Gray if.vi"("Boolean"=w312) -> ("Disabled"=w311:T8)
        n122 = property on="OK" class="Bool"("DisabledEnum"=w311) -> ()  [unwired: 2 in, 2 out]
        n123 = property on="Project" class="CmbBox"("Visible"=w310) -> ()  [unwired: 2 in, 2 out]
      }
      frame "UI: Display Projects" {
        n124 = Unbundle By Name(w340) -> ("Projects"=w339:cluster{"Name":string, "Path":path}[])
        n125 = for {
          tunnel: w339 -> [w343] mode=indexing
          tunnel: [w342] -> w338 mode=indexing
          n126 = Unbundle By Name(w343) -> ("Name"=w342:string)
        }
        n127 = property on="Project" class="CmbBox"("Strings[]"=w338, "Value"="") -> ()  [unwired: 2 in, 2 out]
      }
      frame "---------- Macro ----------" {
        # "Do not put any code in this frame.\n(It is a separator no-op. You can make a copy of this frame to create a new Macro frame)"
      }
      frame "Macro: Initialize" {
        w346 = "Data: Initialize\nInitialize Core Data\nUI: Initialize\nUI: Interlocks\nUI: Front Panel State >> Open"  # Data: Initialize Initialize Core Data UI: Initialize UI: Interlocks UI: Front Panel State >> Open
        # "Initialization Macro\n(This is called once, when the VI starts)"
        n128 = call "Enqueue Multiple States.vi"("State(s) at Front"=w346, "queue in"=w348) -> ()  [unwired: 13 in, 1 out]
      }
      frame "Macro: Exit" {
        # "Exit Macro\n(This is called once, when the VI exits)"
        n129 = Unbundle By Name(w357) -> ("Core.Close Panel on Exit?"=w356:bool)
        n130 = Select(t="UI: Front Panel State >> Close\n", s=w356, f="") -> (s? t:f=w353:string)
        n131 = Concatenate Strings("UI: Uninitialize\n", w353, "Data: Cleanup\nExit") -> (w351:string)
        n132 = call "Enqueue Multiple States.vi"("State(s) at Front"=w351, "queue in"=w358) -> ()  [unwired: 13 in, 1 out]
      }
      frame "---------- Timer ----------" {
        # "Template Separator\n(You can make a copy of, or modify, this frame)"
      }
      frame "Timer: Reset" {
        n133 = call "Timer FGV.vi"("Mode"=FGV_Actions."Write", "error in (no error)"=w366, "Timer Value (s)"=5.0) -> ("error out"=w365:errorcluster)  [unwired: 6 in, 2 out]
      }
      frame "Timer: Poll" {
        n134 = call "Timer FGV.vi"("Mode"=FGV_Actions."Read", "error in (no error)"=w375) -> ("error out"=w374:errorcluster, "Expired?"=w370:bool)  [unwired: 7 in, 1 out]
        n135 = Select(t="Data: Save Hotkey\nUI: Display Hotkeys", s=w370, f="UI: Listen") -> (s? t:f=w367:string)
        n136 = call "Enqueue Multiple States.vi"("queue in"=w373, "State(s) at Back"=w367) -> ()  [unwired: 13 in, 1 out]
      }
    }
  }
  n137 = Merge Errors(w14, w13) -> (w15:errorcluster)
  n138 = Unbundle By Name(w3) -> ("App Ref"=→"App Ref":refnum<vi>, "OK?"=→"OK?":bool)
  n139 = Release Queue(queue=w9, error in (no error)=w15) -> (error out=→"error out":errorcluster)  [unwired: 1 in, 2 out]
